vi "cluster_strict_types_to_strings.vi"(8 "error in (no error)":errorcluster, 9 "Controls[] (strings)":refnum<vi>[](array[refnum]), 10 "Controls[]":refnum<vi>[](array[refnum])) -> (0 "error out":errorcluster)   [LabVIEW 2018]
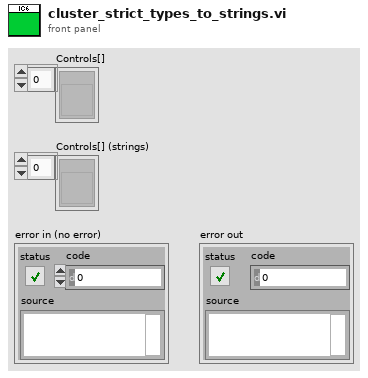
[diagram p1: front panel]
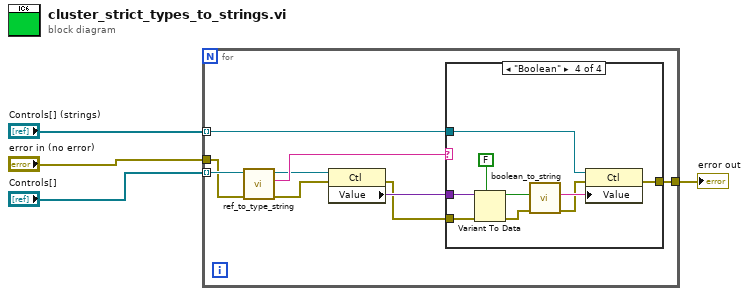
[diagram p0: block diagram]
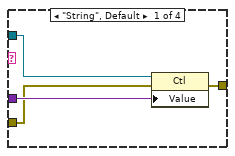
[diagram p2: hidden frame]
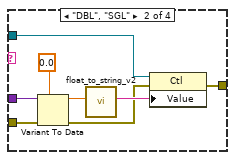
[diagram p3: hidden frame]
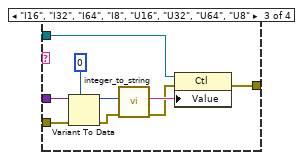
[diagram p4: hidden frame]
diagram:
  n1 = for {
    tunnel: "Controls[] (strings)" -> [w5] mode=indexing
    tunnel: "Controls[]" -> [w12] mode=indexing
    tunnel: "error in (no error)" -> [w11]
    tunnel: [w13] -> w4
    n2 = call "ref_to_type_string.vi"("error in (no error)"=w11, "Control ref in"=w12) -> ("error out"=w10:errorcluster, "Type String"=w9:string, "Control ref out"=w8:refnum<vi>)  [unwired: 7 in]
    n3 = property class="Ctl"(reference=w8, error in=w10) -> (error out=w6:errorcluster, "Value"=w7:variant)  [unwired: 1 out]
    n4 = case shown="\"Boolean\"" w9 {
      tunnel: [w17 w25 w34 w43] -> w13
      tunnel: w7 -> [w16 w22 w29 w37]
      tunnel: w6 -> [w14 w20 w28 w38]
      tunnel: w5 -> [w15 w18 w31 w42]
      frame "String", Default {
        n5 = property class="Ctl"(reference=w15, error in=w14, "Value"=w16) -> (error out=w17:errorcluster)  [unwired: 1 out]
      }
      frame "DBL", "SGL" {
        n6 = Variant To Data(error in=w20, type=sgl 0.0, Variant=w22) -> (data=w21:sgl, error out=w19:errorcluster)
        n7 = call "float_to_string_v2.vi"("Float"=w21) -> ("String"=w24:string)  [unwired: 10 in]
        n8 = property class="Ctl"(reference=w18, error in=w19, "Value"=w24) -> (error out=w25:errorcluster)  [unwired: 1 out]
      }
      frame "I16", "I32", "I64", "I8", "U16", "U32", "U64", "U8" {
        n9 = Variant To Data(error in=w28, type=0, Variant=w29) -> (data=w27:i32, error out=w26:errorcluster)
        n10 = call "integer_to_string.vi"("error in (no error)"=w26, "number"=w27) -> ("error out"=w32:errorcluster, "String"=w33:string)  [unwired: 8 in]
        n11 = property class="Ctl"(reference=w31, error in=w32, "Value"=w33) -> (error out=w34:errorcluster)  [unwired: 1 out]
      }
      frame "Boolean" {
        n12 = Variant To Data(error in=w38, type=FALSE, Variant=w37) -> (data=w36:bool, error out=w35:errorcluster)
        n13 = call "boolean_to_string.vi"("error in (no error)"=w35, "Boolean"=w36) -> ("error out"=w40:errorcluster, "String"=w41:string)  [unwired: 8 in]
        n14 = property class="Ctl"(reference=w42, error in=w40, "Value"=w41) -> (error out=w43:errorcluster)  [unwired: 1 out]
      }
    }
  }
  "error out" <- w4
